vi "Measure_Pump_Rate.vi"(8 "error in (no error)":errorcluster, 10 "ControlQueue":refnum<queue>, 11 "DAQmxTaksContainer_General in":refnum<class "DAQmxTaksContainer_General.lvclass">) -> (0 "error out":errorcluster, 3 "DAQmxTaksContainer_General out":refnum<class "DAQmxTaksContainer_General.lvclass">)   [LabVIEW 2018, in "DAQmxTaksContainer_General.lvclass"]
uses:
  DAQmxTaksContainer_General.lvclass
  DAQmxTaskAITension_General/DAQmxTaskAIVoltage_General.lvclass
  dependecies/ControlsVIs/Clusters-def/SERVER-Commands.ctl
  dependecies/ControlsVIs/Clusters-def/DAQmx-ELYSE_PumpSpeed.ctl
  dependecies/ControlsVIs/Clusters-def/Standard Command.ctl
  DAQmxTaskAITension_General/DAQmxTaskAIVoltage_General.lvclass/DAQmxTaskAIVoltage_General.ctl
  DAQmxTask.lvclass
  Control/Control-Server/Control-Server.lvclass
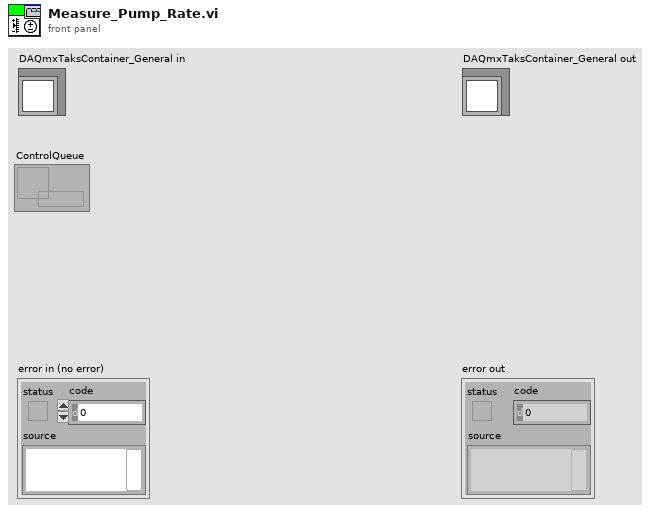
[diagram p1: front panel]
types:
  T1 = typedef "Standard Command.ctl" = cluster{"command":string, "data":variant}
  T2 = typedef "DAQmxTaksContainer_General.lvclass/DAQmx-ELYSE_PumpSpeed.ctl" = cluster{"speed, rpm":dbl}
  T3 = typedef "Control-Server.lvclass/SERVER-Commands.ctl" = string
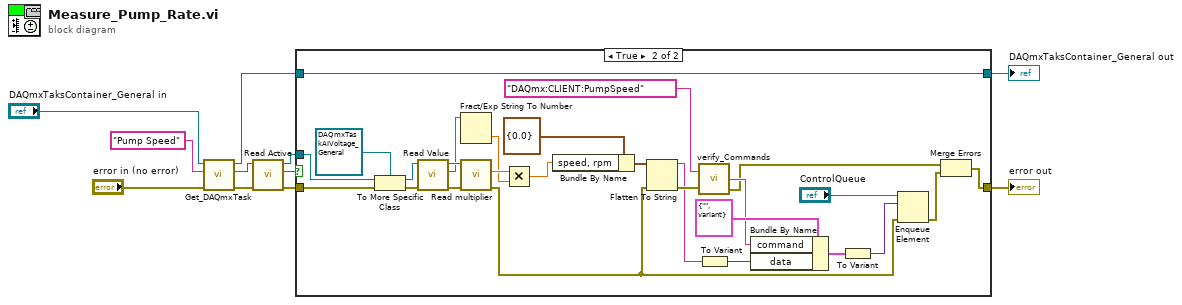
[diagram p0: block diagram]
diagram:
  n1 = call "Get_DAQmxTask.vi"("error in (no error)"="error in (no error)", "Task name"="Pump Speed", "DAQmxTaksContainer_General in"="DAQmxTaksContainer_General in") -> ("error out"=w9:errorcluster, "DAQmx Task"=w8:refnum<class "DAQmxTask.lvclass">, "DAQmxTaksContainer_General out"=w1:refnum<class "DAQmxTaksContainer_General.lvclass">)  [unwired: 6 in]
  n2 = call-dynamic "Read Active.vi"("error in (no error)"=w9, "DAQmxTask in"=w8) -> ("error out"=w4:errorcluster, "Active?"=w7:bool, "DAQmxTask out"=w3:refnum<class "DAQmxTask.lvclass">)  [unwired: 7 in]
  n3 = case shown="True" w7 {
    tunnel: [w13 w14] -> w5
    tunnel: w4 -> [w13 w36]
    tunnel: w3 -> [_ w40]
    tunnel: [w12 w24] -> w2
    tunnel: w1 -> [w12 w24]
    frame False {
    }
    frame True {
      n4 = To More Specific Class(target class=refnum<class "DAQmxTaskAIVoltage_General.lvclass"> refnum ("DAQmxTaskAIVoltage_General.lvclass"), reference=w40, error in=w36) -> (specific class reference=w38:refnum<class "DAQmxTaskAIVoltage_General.lvclass">, error out=w35:errorcluster)
      n5 = call-dynamic "Read Value.vi"("error in (no error)"=w35, "DAQmxTask en entrée"=w38) -> ("error out"=w34:errorcluster, "Data string"=w32:string, "DAQmxTask en sortie"=w37:refnum<class "DAQmxTaskAIVoltage_General.lvclass">)  [unwired: 6 in, 1 out]
      n6 = Fract/Exp String To Number(string=w32) -> (number=w31:dbl)  [unwired: 3 in, 1 out]
      n7 = call "Read multiplier.vi"("error in (no error)"=w34, "DAQmxTaskAIVoltage_General in"=w37) -> ("error out"=w17:errorcluster, "multiplier"=w33:dbl)  [unwired: 7 in, 1 out]
      n8 = Multiply(x=w33, y=w31) -> (x*y=w26:dbl)
      n9 = Bundle By Name(cluster=T2 {"speed, rpm"=0.0} ("OSc:Read"), "speed, rpm"=w26) -> (w23:T2)
      n10 = Flatten To String(anything=w23, error in (no error)=w17) -> (data string=w22:string, error out=w28:errorcluster)  [unwired: 2 in, 1 out]
      n11 = call "verify_Commands.vi"("Command"=T3 "DAQmx:CLIENT:PumpSpeed" ("Commands"), "error in"=w28) -> ("Command out"=w25:string, "error out"=w16:errorcluster)  [unwired: 1 out]
      n12 = To Variant(anything=w22) -> (Variant=w21:variant)
      n13 = Bundle By Name(cluster=T1 {"command"="", "data"=variant} ("input cluster"), "command"=w25, "data"=w21) -> (w19:T1)
      n14 = To Variant(anything=w19) -> (Variant=w18:variant)
      n15 = Enqueue Element(queue="ControlQueue", element=w18, error in (no error)=w17) -> (error out=w15:errorcluster)  [unwired: 1 in, 2 out]
      n16 = Merge Errors(w16, w15) -> (w14:errorcluster)
    }
  }
  "error out" <- w5
  "DAQmxTaksContainer_General out" <- w2
